vi "Pulse Graph Helper.vi"(0 "Puls Times":refnum<vi>[](array[refnum]), 1 "Settings in":refnum<class "Settings.lvclass">, 5 "Exosure (s)":dbl, 9 "Pulse Names":string[](array[string]), 11 "New Dye Name":string, 12 "Selected Dye":i32) -> (3 "Yellow Select":bool, 4 "Graph":cluster{dbl[], dbl[]}[](array[cluster]), 6 "Pulse Sequence":T1(array[cluster]), 8 "# Pulses":i32, 10 "Exosure new (s)":dbl, 15 "Error?":bool)   [LabVIEW 2010, in "Settings.lvclass"]
uses:
  Settings.lvclass
  Settings.lvclass/Settings.ctl
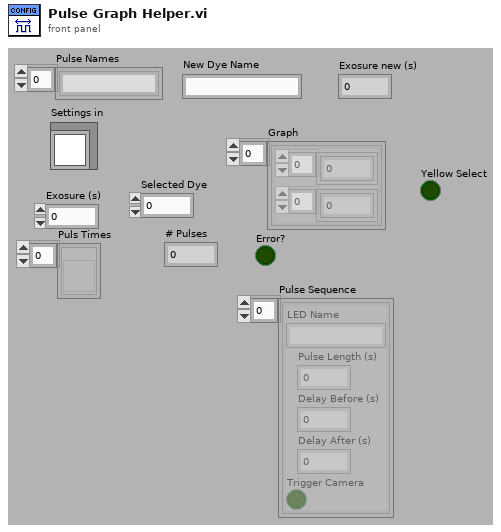
[diagram p1: front panel]
types:
  T1 = cluster{"LED Name":string, "Pulse Length (s)":dbl, "Delay Before (s)":dbl, "Delay After (s)":dbl, "Trigger Camera":bool}[]
  T2 = cluster{"LED Name":string, "Pulse Length (s)":dbl, "Delay Before (s)":dbl, "Delay After (s)":dbl, "Trigger Camera":bool}
  T3 = enum8{"Enabled", "Disabled", "Disabled and Grayed Out"}
  T4 = cluster{"Color":string, "DLL LED Num":i32, "Wavelength":i32, "Counter Name":string, "GRN_YEL":i32, "Yellow Select":i32, "Yellow Select Line":string}[]
  T5 = cluster{"Dye Name":string, "Pulse Sequence":cluster{"LED Name":string, "Pulse Length (s)":dbl, "Delay Before (s)":dbl, "Delay After (s)":dbl, "Trigger Camera":bool}[], "Emission Filter":i16, "Exposure (s)":dbl, "Yellow Select":bool, "# Pulses":i32}[]
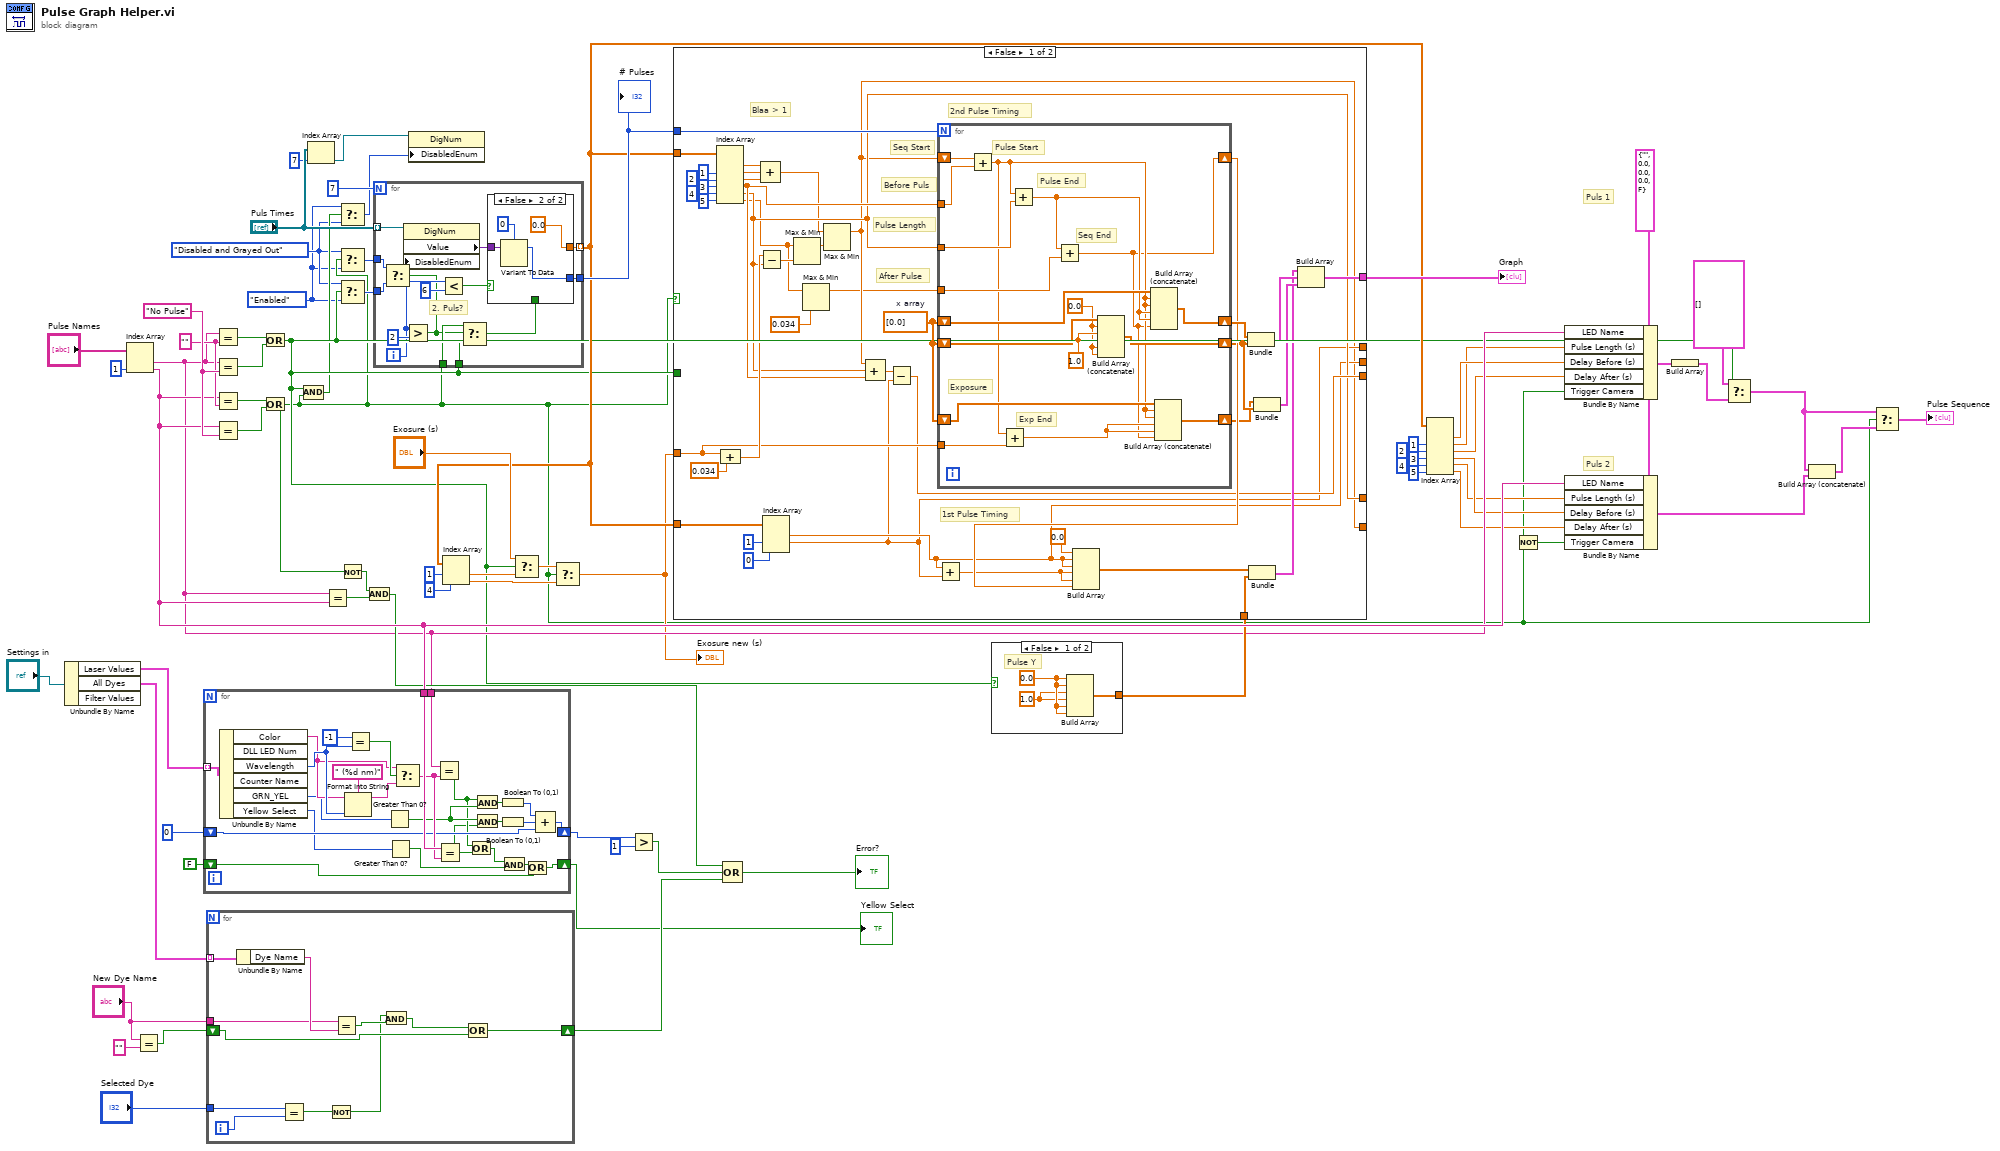
[diagram p0: block diagram]
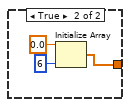
[diagram p2: hidden frame]
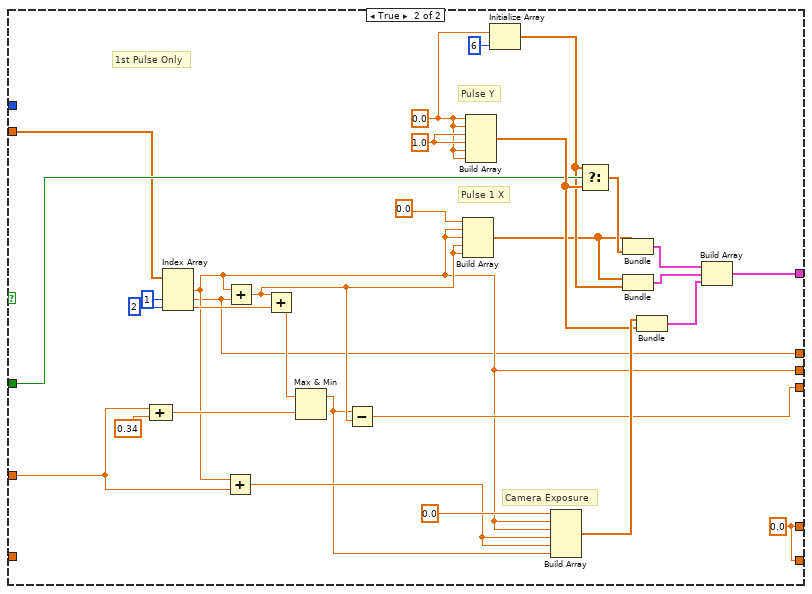
[diagram p3: hidden frame]
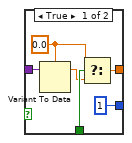
[diagram p4: hidden frame]
diagram:
  w56 = T2 {"LED Name"="", "Pulse Length (s)"=0.0, "Delay Before (s)"=0.0, "Delay After (s)"=0.0, "Trigger Camera"=FALSE} ("element")
  w1 = T3."Enabled" ("Disabled")
  w2 = T3."Disabled and Grayed Out" ("Disabled")
  w68 = "No Pulse" ("y")
  w67 = "" ("y")
  # "Puls 2"
  # "Puls 1"
  n1 = Unbundle By Name("Settings in") -> ("Laser Values"=w41:T4, "All Dyes"=w40:T5)  [unwired: 1 out]
  n2 = Index Array(array="Pulse Names", index #2=1 ("index")) -> (element #1=w30:string, element #2=w48:string)  [unwired: 1 in]
  n3 = Equal?(x="New Dye Name", y="") -> (x = y?=w36:bool)
  n4 = for {
    tunnel: w41 -> [w97] mode=indexing
    tunnel: w30 -> [w90]
    tunnel: w48 -> [w89]
    shift-right: [w80] -> w50
    shift-left: i16 0 -> [w81]
    shift-right: [w73] -> w33
    shift-left: FALSE -> [w72]
    n5 = Unbundle By Name(w97) -> ("Color"=w91:string, "Wavelength"=w92:i32, "GRN_YEL"=w87:i32, "Yellow Select"=w79:i32)  [unwired: 2 out]
    n6 = Format Into String(format string=" (%d nm)", initial string=w91, w92) -> (resulting string=w93:string)  [unwired: 1 in, 1 out]
    n7 = Equal?(x=-1, y=w92) -> (x = y?=w94:bool)
    n8 = Greater Than 0?(x=w87) -> (x > 0?=w86:bool)
    n9 = Greater Than 0?(x=w79) -> (x > 0?=w75:bool)
    n10 = Select(t=w91, s=w94, f=w93) -> (s? t:f=w88:string)
    n11 = Equal?(x=w90, y=w88) -> (x = y?=w78:bool)
    n12 = Equal?(x=w89, y=w88) -> (x = y?=w77:bool)
    n13 = Or(x=w78, y=w77) -> (x .or. y?=w76:bool)
    n14 = And(x=w78, y=w86) -> (x .and. y?=w84:bool)
    n15 = And(x=w86, y=w77) -> (x .and. y?=w85:bool)
    n16 = Boolean To (0,1)(Boolean=w84) -> (0, 1=w83:i16)
    n17 = Boolean To (0,1)(Boolean=w85) -> (0, 1=w82:i16)
    n18 = And(x=w76, y=w75) -> (x .and. y?=w74:bool)
    n19 = Or(x=w74, y=w72) -> (x .or. y?=w73:bool)
    n20 = Compound Arithmetic op=ADD(w83, w82, w81) -> (w80:i16)
  }
  "Yellow Select" <- w33
  n21 = for {
    tunnel: w40 -> [w108] mode=indexing
    tunnel: "New Dye Name" -> [w106]
    shift-right: [w105] -> w39
    shift-left: w36 -> [w104]
    tunnel: "Selected Dye" -> [w102]
    i -> [w103]
    n22 = Unbundle By Name(w108) -> ("Dye Name"=w107:string)
    n23 = Equal?(x=w102, y=w103) -> (x = y?=w101:bool)
    n24 = Not(x=w101) -> (.not. x?=w99:bool)
    n25 = Equal?(x=w106, y=w107) -> (x = y?=w100:bool)
    n26 = And(x=w99, y=w100) -> (x .and. y?=w98:bool)
    n27 = Or(x=w98, y=w104) -> (x .or. y?=w105:bool)
  }
  n28 = Equal?(x=w30, y=w67) -> (x = y?=w66:bool)
  n29 = Equal?(x=w30, y=w68) -> (x = y?=w65:bool)
  n30 = Equal?(x=w48, y=w67) -> (x = y?=w64:bool)
  n31 = Equal?(x=w48, y=w68) -> (x = y?=w63:bool)
  n32 = Or(x=w66, y=w65) -> (x .or. y?=w6:bool)
  n33 = Or(x=w64, y=w63) -> (x .or. y?=w4:bool)
  n34 = Compound Arithmetic op=AND(w6, w4) -> (w3:bool)
  n35 = Index Array(array="Puls Times", index=7) -> (element=w7:refnum<vi>)
  n36 = Equal?(x=w30, y=w48) -> (x = y?=w47:bool)
  n37 = Select(t=w1, s=w3, f=w2) -> (s? t:f=w5:T3)
  n38 = Select(t=w2, s=w4, f=w1) -> (s? t:f=w61:T3)
  n39 = Select(t=w2, s=w6, f=w1) -> (s? t:f=w62:T3)
  n40 = Not(x=w4) -> (.not. x?=w46:bool)
  n41 = And(x=w46, y=w47) -> (x .and. y?=w45:bool)
  n42 = for {
    N: 7 -> [_]
    tunnel: "Puls Times" -> [w123] mode=indexing
    tunnel: [w122] -> w16 mode=indexing
    tunnel: w4 -> [w119]
    tunnel: w62 -> [w110]
    tunnel: w61 -> [w109]
    tunnel: w6 -> [w120]
    tunnel: [w113] -> w32
    i -> [w116]
    # "2. Puls?"
    n43 = Greater?(x=w116, y=2) -> (0:w111:bool)
    n44 = Select(t=w109, s=w111, f=w110) -> (s? t:f=w112:T3)
    n45 = property on="Property Node" class="DigNum"(reference=w123, "DisabledEnum"=w112) -> ("Value"=w117:variant)  [unwired: 1 in, 2 out]
    n46 = Less?(x=w116, y=6) -> (x < y?=w114:bool)
    n47 = Select(t=w119, s=w111, f=w120) -> (s? t:f=w118:bool)
    n48 = case shown="False" w114 {
      tunnel: [w129 0.0 ("t")] -> w122
      tunnel: w118 -> [w128 _]
      tunnel: w117 -> [w127 w133]
      tunnel: [1 ("t") w130] -> w113
      frame True {
        w126 = 0.0 ("t")
        n49 = Variant To Data(Variant=w127, type=w126) -> (data=w125:dbl)  [unwired: 1 in, 1 out]
        n50 = Select(t=w126, s=w128, f=w125) -> (s? t:f=w129:dbl)
      }
      frame False {
        n51 = Variant To Data(Variant=w133, type=0 ("t")) -> (data=w130:i32)  [unwired: 1 in, 1 out]
      }
    }
  }
  "# Pulses" <- w32
  n52 = property on="Property Node" class="DigNum"(reference=w7, "DisabledEnum"=w5) -> ()  [unwired: 1 in, 2 out]
  n53 = Index Array(array=w16, index #1=1 ("index"), index #2=4 ("index")) -> (element #1=w13:dbl, element #2=w12:dbl)
  n54 = Select(t="Exosure (s)", s=w6, f=w13) -> (s? t:f=w20:dbl)
  n55 = Select(t=w20, s=w4, f=w12) -> (s? t:f=w11:dbl)
  "Exosure new (s)" <- w11
  n56 = Greater?(x=w50, y=i16 1) -> (0:w44:bool)
  n57 = Compound Arithmetic op=OR(w45, w44, w39) -> (→"Error?":bool)
  n58 = case shown="False" w6 {
    tunnel: [w134 w138] -> w31
    frame False {
      w135 = 1.0 ("Delay After (s) 2")
      w136 = 0.0 ("Delay After (s) 2")
      # "Pulse Y"
      n59 = Build Array(w136, w136, w135, w135, w136, w136) -> (w134:dbl[])
    }
    frame True {
      n60 = Initialize Array(0.0 ("element"), 6 ("dimension size")) -> (w138:dbl[])
    }
  }
  n61 = case shown="False" w4 {
    tunnel: [w168 w221] -> w71
    tunnel: w11 -> [w165 w217]
    tunnel: [w143 w201] -> _
    tunnel: [w152 w209] -> _
    tunnel: w6 -> [_ w208]
    tunnel: w16 -> [w176 w207]
    tunnel: w32 -> [w169 _]
    tunnel: w16 -> [w162 _]
    tunnel: w31 -> [w155 _]
    tunnel: [w149 w201] -> _
    tunnel: [w148 w200] -> _
    tunnel: [w147 w199] -> _
    frame False {
      w166 = dbl[] [0.0]  # x array
      # "Seq Start"
      # "1st Pulse Timing"
      # "2nd Pulse Timing"
      # "After Pulse"
      # "Pulse Length"
      # "Before Puls"
      # "Blaa > 1"
      n62 = Index Array(array=w176, index #2=1 ("index"), index #3=2 ("index"), index #4=3 ("index"), index #5=4 ("index"), index #6=5 ("index")) -> (element #1=w173:dbl, element #2=w175:dbl, element #3=w174:dbl, element #4=w154:dbl, element #5=w149:dbl, element #6=w141:dbl)  [unwired: 1 in]
      n63 = Compound Arithmetic op=ADD(w165, 0.034 ("Delay After (s) 2")) -> (w171:dbl)
      n64 = Subtract(x=w171, y=w149) -> (x-y=w170:dbl)
      n65 = Compound Arithmetic op=ADD(w173, w175, w174) -> (w144:dbl)
      n66 = Index Array(array=w162, index #2=1 ("index"), index #3=0 ("index")) -> (element #1=w148:dbl, element #2=w147:dbl)  [unwired: 1 in, 1 out]
      n67 = Max & Min(x=w141, y=w170) -> (max(x,y)=w145:dbl)  [unwired: 1 out]
      n68 = Max & Min(x=w141, y=0.034 ("Delay After (s) 2")) -> (max(x,y)=w142:dbl)  [unwired: 1 out]
      n69 = Max & Min(x=w144, y=w145) -> (max(x,y)=w143:dbl)  [unwired: 1 out]
      n70 = Compound Arithmetic op=ADD(w143, w149, w154) -> (w153:dbl)
      n71 = Subtract(x=w153, y=w147) -> (x-y=w152:dbl)
      n72 = Add(x=w148, y=w147) -> (x+y=w158:dbl)
      n73 = for {
        N: w169 -> [_]
        shift-right: [w182] -> w159
        shift-left: w143 -> [w198]
        tunnel: w142 -> [w195]
        tunnel: w154 -> [w197]
        tunnel: w149 -> [w196]
        shift-right: [w192] -> w164
        shift-left: w166 -> [w194]
        shift-right: [w190] -> w151
        shift-left: w166 -> [w191]
        shift-right: [w186] -> w150
        shift-left: w166 -> [w187]
        tunnel: w165 -> [w185]
        w189 = 1.0 ("x+y")
        w188 = 0.0 ("x+y")
        # "Exp End"
        # "Exposure"
        # "Seq End"
        # "Pulse End"
        # "Pulse Start"
        n74 = Add(x=w198, y=w197) -> (x+y=w184:dbl)
        n75 = Add(x=w184, y=w185) -> (x+y=w183:dbl)
        n76 = Add(x=w184, y=w196) -> (x+y=w193:dbl)
        n77 = Add(x=w193, y=w195) -> (x+y=w182:dbl)
        n78 = Build Array (concatenate)(w191, w188, w189, w189, w188, w188) -> (w190:dbl[])
        n79 = Build Array (concatenate)(w194, w184, w184, w193, w193, w182) -> (w192:dbl[])
        n80 = Build Array (concatenate)(w187, w184, w184, w183, w183, w182) -> (w186:dbl[])
      }
      n81 = Build Array(0.0 ("x+y"), w148, w148, w158, w158, w159) -> (w157:dbl[])
      n82 = Bundle("x array"=w164, "x array"=w151) -> (w167:cluster{"x array":dbl[], "x array":dbl[]})  [unwired: 1 in]
      n83 = Bundle(w157, w155) -> (w156:cluster{dbl[], dbl[]})  [unwired: 1 in]
      n84 = Bundle("x array"=w150, "x array"=w151) -> (w163:cluster{"x array":dbl[], "x array":dbl[]})  [unwired: 1 in]
      n85 = Build Array(w156, w167, w163) -> (w168:cluster{"x array":dbl[], "x array":dbl[]}[])
    }
    frame True {
      w201 = 0.0 ("t")
      w225 = 1.0 ("Delay After (s) 2")
      w215 = 0.0 ("Delay After (s) 2")
      # "1st Pulse Only"
      # "Camera Exposure"
      # "Pulse Y"
      # "Pulse 1 X"
      n86 = Compound Arithmetic op=ADD(w217, 0.34 ("Delay After (s) 2")) -> (w206:dbl)
      n87 = Index Array(array=w207, index #2=1 ("index"), index #3=2 ("index")) -> (element #1=w200:dbl, element #2=w199:dbl, element #3=w226:dbl)  [unwired: 1 in]
      n88 = Add(x=w200, y=w217) -> (x+y=w216:dbl)
      n89 = Add(x=w200, y=w199) -> (x+y=w210:dbl)
      n90 = Add(x=w210, y=w226) -> (x+y=w202:dbl)
      n91 = Max & Min(x=w202, y=w206) -> (max(x,y)=w203:dbl)  [unwired: 1 out]
      n92 = Subtract(x=w203, y=w210) -> (x-y=w209:dbl)
      n93 = Build Array(0.0 ("Delay After (s) 2"), w200, w200, w210, w210) -> (w204:dbl[])
      n94 = Build Array(w215, w215, w225, w225, w215, w215) -> (w213:dbl[])
      n95 = Initialize Array(w215, 6 ("dimension size")) -> (w205:dbl[])
      n96 = Build Array(0.0 ("Delay After (s) 2"), w200, w200, w216, w216, w203) -> (w220:dbl[])
      n97 = Select(t=w205, s=w208, f=w213) -> (s? t:f=w212:dbl[])
      n98 = Bundle(w204, w212) -> (w224:cluster{dbl[], dbl[]})  [unwired: 1 in]
      n99 = Bundle(w204, w205) -> (w223:cluster{dbl[], dbl[]})  [unwired: 1 in]
      n100 = Bundle(w220, w213) -> (w219:cluster{dbl[], dbl[]})  [unwired: 1 in]
      n101 = Build Array(w224, w223, w219) -> (w221:cluster{dbl[], dbl[]}[])
    }
  }
  "Graph" <- w71
  n102 = Index Array(array=w16, index #2=1 ("index"), index #3=2 ("index"), index #4=3 ("index"), index #5=4 ("index"), index #6=5 ("index")) -> (element #1=w24:dbl, element #2=w18:dbl, element #3=w23:dbl, element #4=w22:dbl, element #5=w19:dbl, element #6=w21:dbl)  [unwired: 1 in]
  n103 = Not(x=w4) -> (.not. x?=w60:bool)
  n104 = Bundle By Name(cluster=w56, "LED Name"=w30, "Pulse Length (s)"=w18, "Delay Before (s)"=w24, "Delay After (s)"=w23, "Trigger Camera"=w4) -> (w58:T2)
  n105 = Bundle By Name(cluster=w56, "LED Name"=w48, "Pulse Length (s)"=w19, "Delay Before (s)"=w22, "Delay After (s)"=w21, "Trigger Camera"=w60) -> (w53:T2)
  n106 = Build Array(w58) -> (w57:T1)
  n107 = Select(t=T1 [], s=w6, f=w57) -> (s? t:f=w55:T1)
  n108 = Build Array (concatenate)(w55, w53) -> (w54:T1)
  n109 = Select(t=w55, s=w4, f=w54) -> (s? t:f=→"Pulse Sequence":T1)
